vi "Normal Stream.vi"(8 "error in (no error)":errorcluster, 9 "Stream in":refnum<k5>, 11 "Streamable Response in":refnum<class "Streamable Response.lvclass">) -> (0 "error out":errorcluster, 1 "Stream out":refnum<k5>, 3 "Streamable Response out":refnum<class "Streamable Response.lvclass">)   [LabVIEW 2020, in "HTTP Utils.lvlib" / "Streamable Response.lvclass"]
uses:
  Streamable Response.lvclass
  lv-stream/stream/Stream/Stream.lvclass/Stream.ctl
  lv-stream/stream/Stream/Dispatch Sniffer Data.vi
  lv-stream/stream/Stream/Prepared.vi
  lv-stream/stream/Endpoint/Cast Sniffer Callback.vi
  lv-stream/stream/Error Bad State.vi
  <vilib>/Utility/error.llb/Error Cluster From Error Code.vi
  lv-stream/stream/Stream/Stream.lvclass
  Streamable Response.lvclass/Streamable Response.ctl
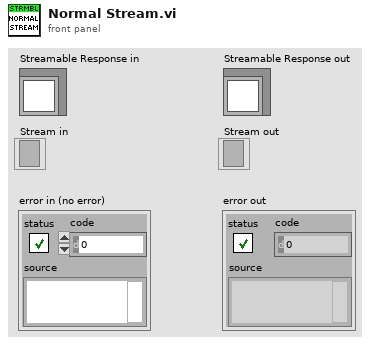
[diagram p1: front panel]
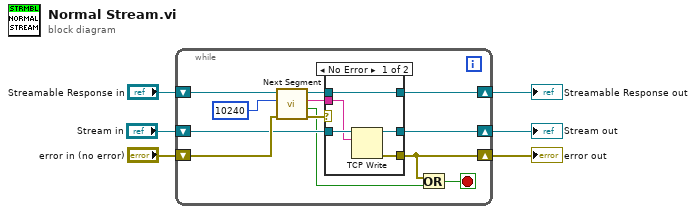
[diagram p0: block diagram]
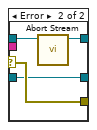
[diagram p2: hidden frame]
diagram:
  n1 = while {
    shift-right: [w13] -> w1
    shift-left: "Streamable Response in" -> [w18]
    shift-right: [w9] -> w3
    shift-left: "error in (no error)" -> [w16]
    shift-right: [w10] -> w2
    shift-left: "Stream in" -> [w12]
    stop <- w7 stop-if-true
    n2 = call-dynamic "Next Segment.vi"("error in (no error)"=w16, "Count"=10240, "Streamable Response in"=w18) -> ("error out"=w15:errorcluster, "Last?"=w8:bool, "Data"=w11:string, "Streamable Response out"=w14:refnum<class "Streamable Response.lvclass">)  [unwired: 5 in]
    n3 = case shown="No Error" w15 {
      selector: w15 -> [_ w25]
      tunnel: w14 -> [w23 w27]
      tunnel: [w23 w26] -> w13
      tunnel: [w21 w25] -> w9
      tunnel: w12 -> [w20 w24]
      tunnel: w11 -> [w19 _]
      tunnel: [w22 w24] -> w10
      frame No Error {
        n4 = TCP Write(connection ID=w20, data in=w19) -> (connection ID out=w22:refnum<k5>, error out=w21:errorcluster)  [unwired: 2 in, 1 out]
      }
      frame Error {
        n5 = call-dynamic "Abort Stream.vi"("Streamable Response in"=w27) -> ("Streamable Response out"=w26:refnum<class "Streamable Response.lvclass">)  [unwired: 9 in, 1 out]
      }
    }
    n6 = Or(x=w9, y=w8) -> (x .or. y?=w7:bool)
  }
  "error out" <- w3
  "Streamable Response out" <- w1
  "Stream out" <- w2
